vi "CH375_Open.vi"(8 "Error In":errorcluster caption="错误输入") -> (0 "Error Out":errorcluster caption="错误输出")   [LabVIEW 2020]
uses:
  <vilib>/Utility/config.llb/Read Key (Double).vi
  Global_CH375.vi
  <vilib>/Utility/config.llb/NI_LVConfig.lvlib
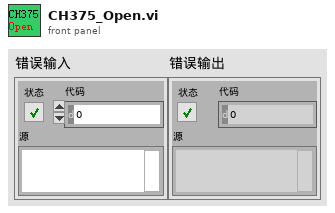
[diagram p1: front panel]
types:
  T1 = typedef "NI_LVConfig.lvlib/Config Data RefNum.ctl" = refnum<k1>
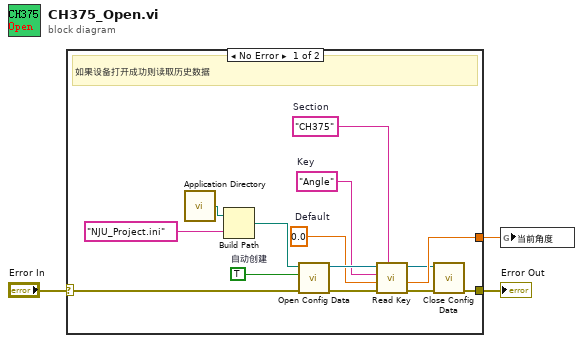
[diagram p0: block diagram]
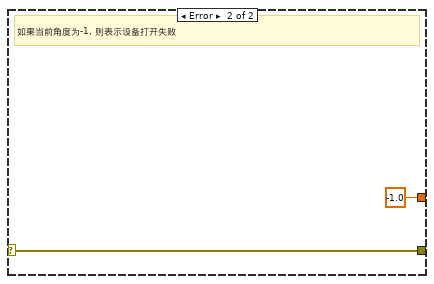
[diagram p2: hidden frame]
diagram:
  n1 = case shown="No Error" "Error In" {
    selector: "Error In" -> [w4 w18]
    tunnel: [w9 -1.0] -> w3
    tunnel: [w6 w18] -> w1
    frame No Error {
      w12 = 0.0  # Default
      w11 = "Angle"  # Key
      w13 = "CH375"  # Section
      w10 = TRUE  # 自动创建
      # "如果设备打开成功则读取历史数据"
      n2 = call <vilib>:"Application Directory.vi"() -> ("Application Directory"=w14:path)
      n3 = Build Path(base path=w14, name or relative path="NJU_Project.ini") -> (appended path=w16:path)
      n4 = call <vilib>:"Open Config Data.vi"("error in (no error)"=w4, "create file if necessary (T)"=w10, "configuration file path"=w16) -> ("error out"=w8:errorcluster, "refnum"=w17:T1)  [unwired: 6 in, 1 out]
      n5 = call-poly <vilib>:"Read Key.vi"("section"=w13, "error in (no error)"=w8, "default value"=w12, "key"=w11, "refnum"=w17) -> ("error out"=w7:errorcluster, "value"=w9:dbl, "refnum out"=w5:T1)  [unwired: 3 in, 1 out]
      n6 = call <vilib>:"Close Config Data.vi"("error in (no error)"=w7, "refnum"=w5) -> ("error out"=w6:errorcluster)  [unwired: 8 in, 1 out]
    }
    frame Error {
      # "如果当前角度为-1, 则表示设备打开失败"
    }
  }
  "Error Out" <- w1
  n7 = global write "Global_CH375.vi" "当前角度"(w3) -> ()
